vi "Get Descriptions.vi"(0 "Robot Arm in":refnum<class "Robot Arm.lvclass">, 11 "error in (no error)":errorcluster) -> (4 "Robot Arm out":refnum<class "Robot Arm.lvclass">, 6 "Name":string, 8 "Comment":string, 10 "Manufacturer":string, 15 "error out":errorcluster)   [LabVIEW 2013, in "Robot Arm.lvclass"]
uses:
  Robot Arm.lvclass
  Robot Arm.lvclass/Robot Arm.ctl
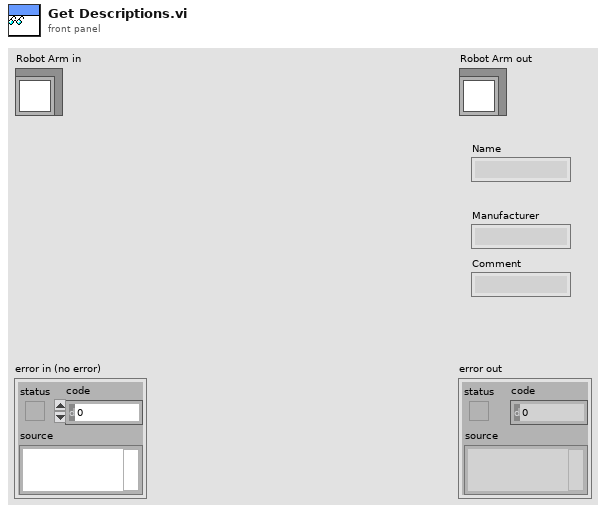
[diagram p1: front panel]
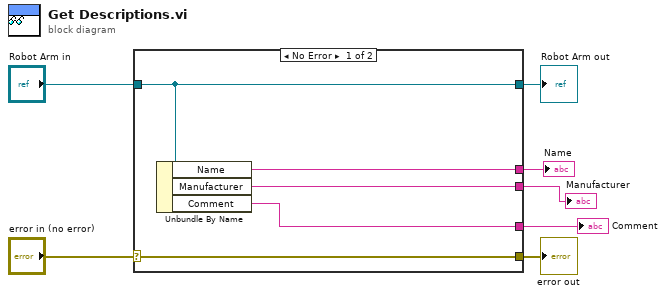
[diagram p0: block diagram]
diagram:
  n1 = case shown="No Error" "error in (no error)" {
    selector: "error in (no error)" -> [w12 w13]
    tunnel: [w12 w13] -> w6
    tunnel: [w11 w14] -> w4
    tunnel: "Robot Arm in" -> [w11 w14]
    tunnel: [w10 _] -> w3
    tunnel: [w9 _] -> w2
    tunnel: [w8 _] -> w1
    frame No Error {
      n2 = Unbundle By Name(w11) -> ("Name"=w10:string, "Manufacturer"=w9:string, "Comment"=w8:string)
    }
    frame Error {
    }
  }
  "error out" <- w6
  "Robot Arm out" <- w4
  "Name" <- w3
  "Manufacturer" <- w2
  "Comment" <- w1
